vi "Keithley6487 Bkg Corr.vi"(8 "error in":errorcluster, 9 "ZC Before":bool, 10 "ZC Toggle":bool, 11 "VISA in":refnum<visa-resource-name>="COM3") -> (0 "error out":errorcluster, 2 "ZC After":bool, 3 "VISA out":refnum<visa-resource-name>)   [LabVIEW 2018]
panel:
  in  "Turn ZC Off":string
  in  "Turn ZC On":string
  in  "Query ZC":string=":TRIG:COUN 1;:SYST:ZCH 1;:CURR:RANG 2E-9;:INIT;:SYST:ZCOR:ACQ;:SYST:ZCH 0;:SYST:ZCOR 1;:CURR:RANG:AUTO 1;"
  # "Error out reports Serial I/O errors.\n\nKeithley Error reports error messages returned by the Keithley 6485 picoAmmeter.  Currently, only overvoltage and invalid data errors are supported by this VI."
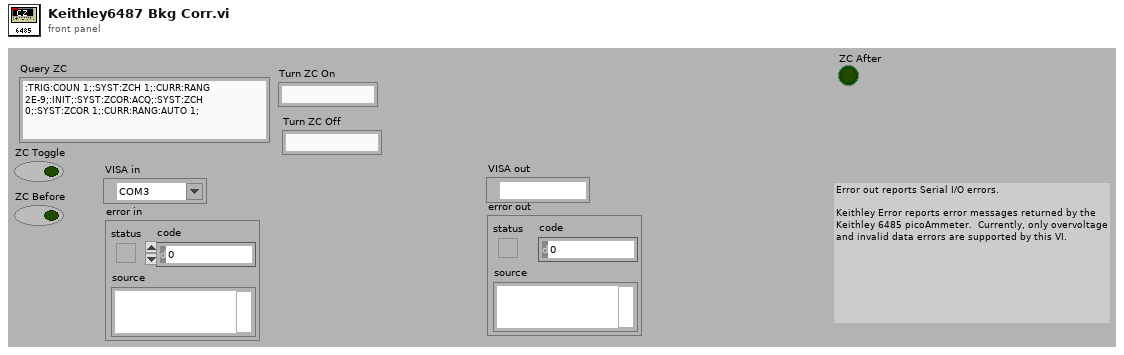
[diagram p1: front panel]
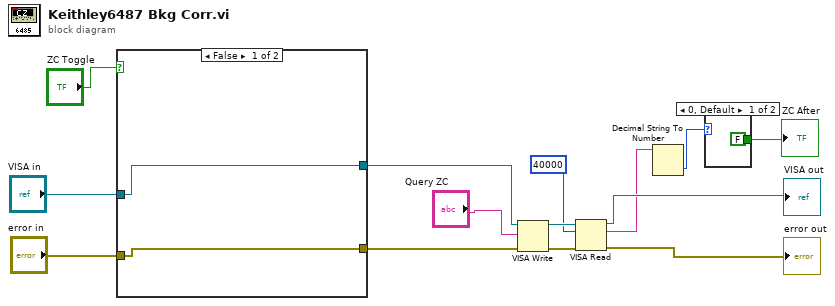
[diagram p0: block diagram]
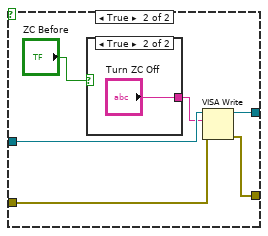
[diagram p2: hidden frame]
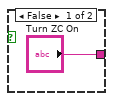
[diagram p3: hidden frame]
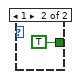
[diagram p4: hidden frame]
diagram:
  n1 = case shown="False" "ZC Toggle" {
    tunnel: [w15 w21] -> w4
    tunnel: [w16 w20] -> w3
    tunnel: "VISA in" -> [w16 w19]
    tunnel: "error in" -> [w15 w18]
    frame False {
    }
    frame True {
      n2 = case shown="True" "ZC Before" {
        tunnel: ["Turn ZC On" "Turn ZC Off"] -> w17
        frame False {
        }
        frame True {
        }
      }
      n3 = VISA Write(VISA resource name=w19, write buffer=w17, error in (no error)=w18) -> (VISA resource name out=w20:refnum<visa-resource-name>, error out=w21:errorcluster)  [unwired: 1 out]
    }
  }
  n4 = VISA Write(VISA resource name=w3, write buffer="Query ZC", error in (no error)=w4) -> (VISA resource name out=w13:refnum<visa-resource-name>, error out=w12:errorcluster)  [unwired: 1 out]
  n5 = VISA Read(VISA resource name=w13, byte count=u32 40000, error in (no error)=w12) -> (VISA resource name out=→"VISA out":refnum<visa-resource-name>, read buffer=w8:string, error out=→"error out":errorcluster)  [unwired: 1 out]
  n6 = Decimal String To Number(string=w8) -> (number=w7:i32)  [unwired: 2 in, 1 out]
  n7 = case shown="0, Default" w7 {
    tunnel: [FALSE TRUE] -> w6
    frame 0, Default {
    }
    frame 1 {
    }
  }
  "ZC After" <- w6
